vi "OldCombinedPythonIDE.vi"(7 "Python version":string="3.9", 11 "Port":string) -> ()   [LabVIEW 2020]
panel:
  out "Script":string
  in  "Example Codes":u16(ring) items=["backpack.py", "Backpack_Demo.py", "Battery.py", "Buttons.py", "Display.py", "Image.py", "LED.py", "Motion.py", "Motor.py", "Sound.py"]
  out "Library":string="Loading...."
  in  "SPIKE Codes":u16(ring) items=["boot.py", "main.py", "version.py", "rogers.py", "backpack.py"]
  out "S_Library":string="Loading..."
  in  "Name":string="code.py"
  in  "Save SPIKE":bool
  in  "Save PC":bool
  in  "Python Code":string
  out "Console":string
  in  "stop":bool
  in  "Ctrl C":bool
  in  "run":bool
  # "PyVIEW IDE\nversion 0.1b01"
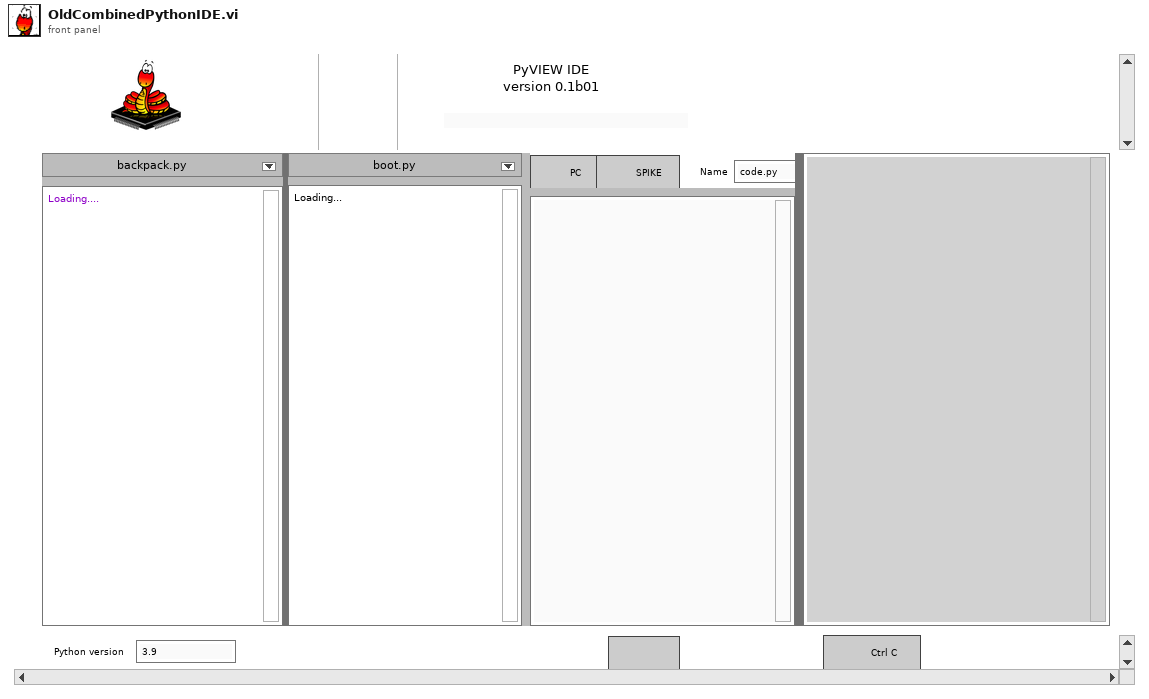
[diagram p1: front panel]
types:
  T1 = typedef "PythonCtrl.ctl" = cluster{"session":refnum<k35>, "PyPath":path, "Processor":enum16{"SPIKE", "Pi", "Pi_ssh"}}
  T2 = typedef "eventvkey.ctl" = enum16{"ASCII", "Enter", "Return", "Shift", "Ctrl", "Alt", "Cmd", "Opt", "Caps", "NumLock", "Clear", "Break", "Up", "Down", "Left", "Right", "Insert", "Delete", "Home", "End", "PageUp", "PageDown", "Escape", "Help", "Pause", "ScrollLock", "F1", "F2", "F3", "F4", "F5", "F6", "F7", "F8", "F9", "F10", "F11", "F12", "F13", "F14", "F15", "F16", "F17", "F18", "F19", "F20", "F21", "F22", "F23", "F24", "Play", "VolumeUp", "VolumeDown", "Mute", "Two Byte Char"}
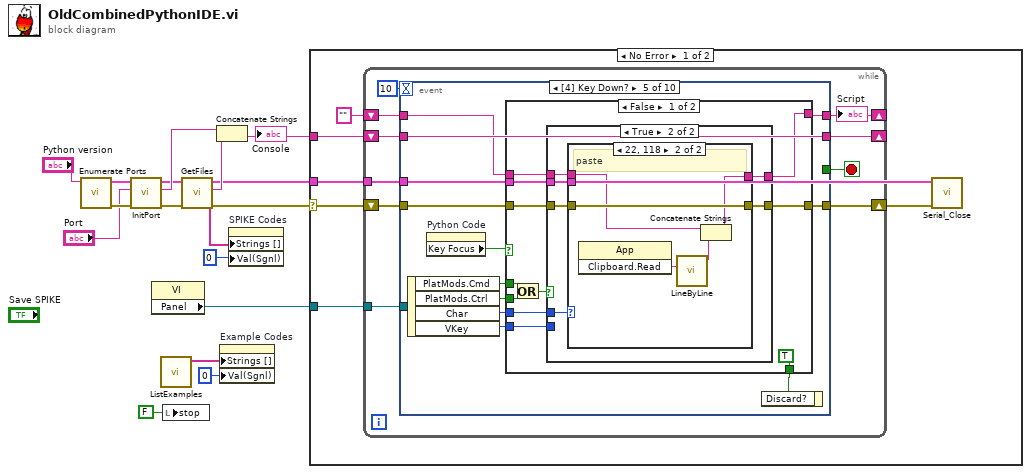
[diagram p0: block diagram]
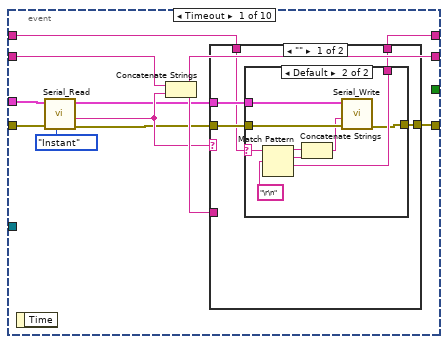
[diagram p2: hidden frame]
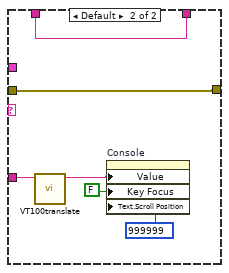
[diagram p4: hidden frame]
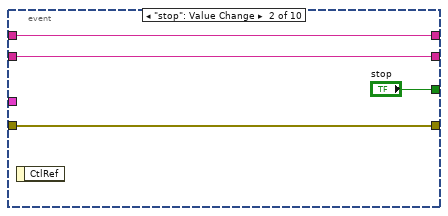
[diagram p5: hidden frame]
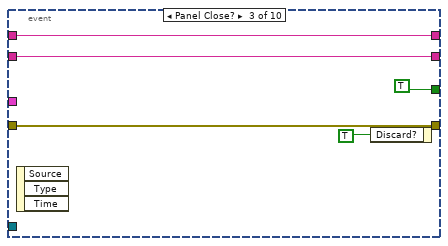
[diagram p6: hidden frame]
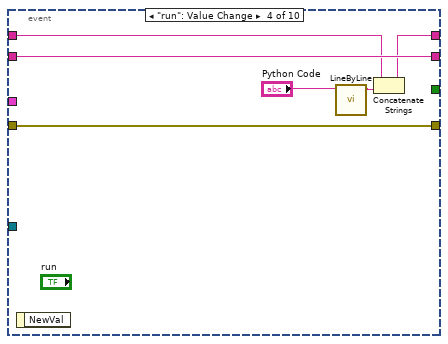
[diagram p7: hidden frame]
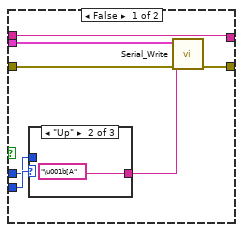
[diagram p8: hidden frame]
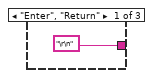
[diagram p9: hidden frame]
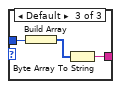
[diagram p10: hidden frame]
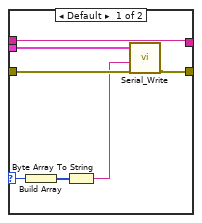
[diagram p11: hidden frame]
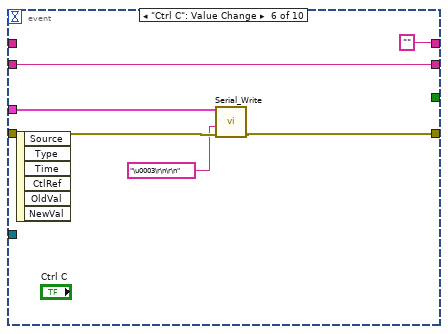
[diagram p14: hidden frame]
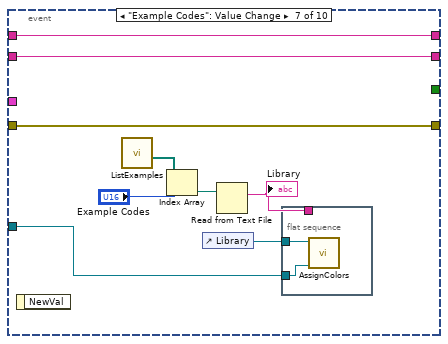
[diagram p15: hidden frame]
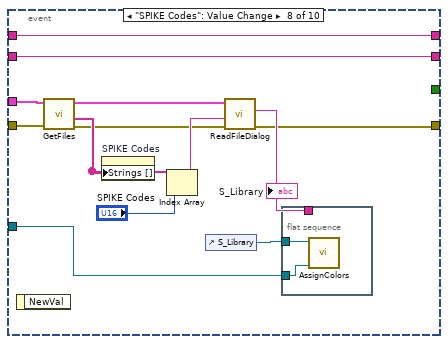
[diagram p16: hidden frame]
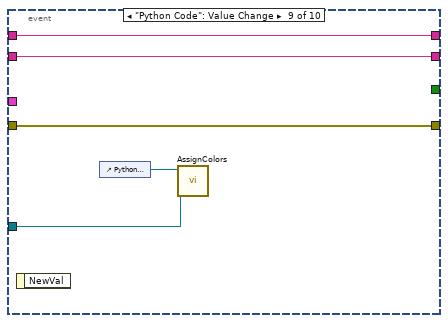
[diagram p17: hidden frame]
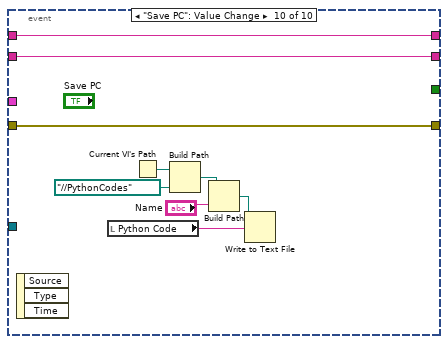
[diagram p18: hidden frame]
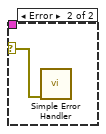
[diagram p19: hidden frame]
diagram:
  n1 = call "Enumerate Ports.vi"("Python version"="Python version") -> ("error out"=w15:errorcluster, "Python"=w9:T1)  [unwired: 6 in, 3 out]
  n2 = call "InitPort.vi"("error in (no error)"=w15, "Port"="Port", "Python"=w9) -> ("error out"=w7:errorcluster, "Console"=w8:string, "Python out"=w4:T1)  [unwired: 6 in]
  n3 = property class="VI"() -> ("Panel"=w10:refnum<vi>)  [unwired: 2 in, 2 out]
  n4 = call "ListExamples.vi"() -> ("filenames"=w11:string[])  [unwired: 7 in, 4 out]
  n5 = local write "stop"(FALSE ("stop")) -> ()
  n6 = call "GetFiles.vi"("error in (no error)"=w7, "Python"=w4) -> ("error out"=w6:errorcluster, "Python files"=w3:string[], "String"=w5:string)  [unwired: 6 in, 1 out]
  n7 = Concatenate Strings(w8, w5) -> (w1:string)
  "Console" <- w1
  n8 = property on="Example Codes" class="Ring (strict)"("Strings []"=w11, "Val(Sgnl)"=u16 0 ("Value (Signaling)")) -> ()  [unwired: 2 in, 2 out]
  n9 = property on="SPIKE Codes" class="Ring (strict)"("Strings []"=w3, "Val(Sgnl)"=u16 0 ("Value (Signaling)")) -> ()  [unwired: 2 in, 2 out]
  n10 = case shown="No Error" w6 {
    selector: w6 -> [w21 w181]
    tunnel: w10 -> [w22 _]
    tunnel: w1 -> [w19 _]
    tunnel: w4 -> [w18 _]
    frame No Error {
      n11 = while {
        shift-right: [w31] -> _
        shift-left: w19 -> [w32]
        shift-right: [w27] -> w17
        shift-left: w21 -> [w28]
        tunnel: w22 -> [w26]
        shift-right: [w24] -> _
        shift-left: "" -> [w25]
        tunnel: w18 -> [w23]
        stop <- w30 stop-if-true
        n12 = event shown="[4] Key Down?" {
          selector: _ -> [_ _ _ _ _ _ _ _ _ _]
          dyn-events: _ -> [_ _ _ _ _ _ _ _ _ _]
          timeout: 10 -> [_ _ _ _ _ _ _ _ _ _]
          tunnel: w23 -> [w34 _ _ _ w91 w140 _ w157 _ _]
          tunnel: w32 -> [w42 w67 w73 w79 w90 w141 w147 w164 w171 w179]
          tunnel: [w41 w67 w73 w79 w90 w141 w147 w164 w171 w179] -> w31
          tunnel: [_ "stop" TRUE ("stop") _ _ _ _ _ _ _] -> w30
          tunnel: w28 -> [w37 w66 w72 w78 w84 w139 w146 w159 w170 w178]
          tunnel: [w40 w66 w72 w78 w85 w137 w146 w153 w170 w178] -> w27
          tunnel: w26 -> [_ _ _ _ _ _ w145 w163 w168 _]
          tunnel: [w39 w65 w69 w76 w80 "" w142 w162 w167 w180] -> w24
          tunnel: w25 -> [w38 w65 w69 w77 w81 _ w142 w162 w167 w180]
          event Timeout {
            n13 = event-data() -> ()  [unwired: 1 in, 1 out]
            n14 = call "Serial_Read.vi"("Task"=enum16{"Instant", "All"}."Instant", "error in (no error)"=w37, "Python"=w34) -> ("error out"=w35:errorcluster, "Text read"=w36:string)  [unwired: 7 in]
            n15 = Concatenate Strings(w42, w36) -> (w41:string)
            n16 = case shown="\"\"" w36 {
              tunnel: w41 -> [_ w64]
              tunnel: w35 -> [w46 w60]
              tunnel: [w45 w60] -> w40
              tunnel: w38 -> [w43 w59]
              tunnel: [w47 w59] -> w39
              tunnel: w34 -> [w44 _]
              frame "" {
                n17 = case shown="Default" w43 {
                  selector: w43 -> [w49 w50]
                  tunnel: [w49 w58] -> w47
                  tunnel: w46 -> [w48 w54]
                  tunnel: [w48 w53] -> w45
                  tunnel: w44 -> [_ w51]
                  frame "" {
                  }
                  frame Default {
                    n18 = Match Pattern(string=w50, regular expression="\r\n") -> (before substring=w56:string, match substring=w55:string, after substring=w58:string)  [unwired: 1 in, 1 out]
                    n19 = Concatenate Strings(w56, w55) -> (w52:string)
                    n20 = call "Serial_Write.vi"("error in (no error)"=w54, "Text to write"=w52, "Python"=w51) -> ("error out"=w53:errorcluster)  [unwired: 8 in]
                  }
                }
              }
              frame Default {
                n21 = call "VT100translate.vi"("Console"=w64) -> ("Console 2"=w62:string)  [unwired: 10 in]
                n22 = property on="Console" class="Str"("Value"=w62, "Key Focus"=FALSE, "Text.Scroll Position"=u32 999999) -> ()  [unwired: 2 in, 2 out]
              }
            }
          }
          event "stop": Value Change {
            n23 = event-data() -> ()  [unwired: 1 in, 1 out]
          }
          event Panel Close? {
            n24 = event-data() -> ()  [unwired: 1 in, 3 out]
            n25 = event-data("Discard?"=TRUE ("stop")) -> ()  [unwired: 1 in, 1 out]
          }
          event "run": Value Change {
            n26 = event-data() -> ()  [unwired: 1 in, 1 out]
            n27 = call "LineByLine.vi"("Python Code"="Python Code") -> ("result string"=w75:string)  [unwired: 10 in]
            n28 = Concatenate Strings(w77, w75) -> (w76:string)
          }
          event Key Down? {
            n29 = event-data() -> ("PlatMods.Cmd"=w86:bool, "PlatMods.Ctrl"=w87:bool, "Char"=w88:i16, "VKey"=w89:T2)  [unwired: 1 in]
            n30 = property on="Python Code" class="Str"() -> ("Key Focus"=w82:bool)  [unwired: 2 in, 2 out]
            n31 = case shown="False" w82 {
              tunnel: w91 -> [w96 _]
              tunnel: w89 -> [w102 _]
              tunnel: w88 -> [w101 w134]
              tunnel: w87 -> [w100 _]
              tunnel: w86 -> [w99 _]
              tunnel: [w94 w135] -> w85
              tunnel: w84 -> [w95 w135]
              tunnel: [TRUE ("Discard?") _] -> w83
              tunnel: w81 -> [w93 w133]
              tunnel: [w92 w133] -> w80
              frame False {
                n32 = Or(x=w99, y=w100) -> (x .or. y?=w98:bool)
                n33 = case shown="True" w98 {
                  tunnel: w102 -> [w109 _]
                  tunnel: w101 -> [w108 w120]
                  tunnel: w96 -> [w107 w119]
                  tunnel: w95 -> [w106 w118]
                  tunnel: [w104 w117] -> w94
                  tunnel: w93 -> [w103 w116]
                  tunnel: [w103 w115] -> w92
                  frame False {
                    n34 = case shown="\"Up\"" w109 {
                      tunnel: w108 -> [_ _ w114]
                      tunnel: ["\r\n" ("replace string (\"\")") "\u001b[A" ("replace string (\"\")") w112] -> w105
                      frame "Enter", "Return" {
                      }
                      frame "Up" {
                      }
                      frame Default {
                        n35 = Build Array(w114) -> (w113:i16[])
                        n36 = Byte Array To String(unsigned byte array=w113) -> (string=w112:string)
                      }
                    }
                    n37 = call "Serial_Write.vi"("error in (no error)"=w106, "Text to write"=w105, "Python"=w107) -> ("error out"=w104:errorcluster)  [unwired: 8 in]
                  }
                  frame True {
                    n38 = case shown="22, 118" w120 {
                      selector: w120 -> [w126 _]
                      tunnel: w119 -> [w125 _]
                      tunnel: w118 -> [w124 w132]
                      tunnel: [w123 w132] -> w117
                      tunnel: w116 -> [w121 w131]
                      tunnel: [w121 w130] -> w115
                      frame Default {
                        n39 = Build Array(w126) -> (w127:i16[])
                        n40 = Byte Array To String(unsigned byte array=w127) -> (string=w122:string)
                        n41 = call "Serial_Write.vi"("error in (no error)"=w124, "Text to write"=w122, "Python"=w125) -> ("error out"=w123:errorcluster)  [unwired: 8 in]
                      }
                      frame 22, 118 {
                        # "paste"
                        n42 = invoke class="App" method="Clipboard.Read"() -> ("Read Clipbrd"=w129:string)  [unwired: 3 in, 2 out]
                        n43 = call "LineByLine.vi"("Python Code"=w129) -> ("result string"=w128:string)  [unwired: 10 in]
                        n44 = Concatenate Strings(w131, w128) -> (w130:string)
                      }
                    }
                  }
                }
              }
              frame True {
                n45 = case shown="1" w134 {
                  frame 0, Default {
                  }
                  frame 1 {
                  }
                }
              }
            }
            n46 = event-data("Discard?"=w83) -> ()  [unwired: 1 in, 1 out]
          }
          event "Ctrl C": Value Change {
            n47 = event-data() -> ()  [unwired: 1 in, 6 out]
            n48 = call "Serial_Write.vi"("error in (no error)"=w139, "Text to write"="\u0003\r\n\r\n" ("function name"), "Python"=w140) -> ("error out"=w137:errorcluster)  [unwired: 8 in]
          }
          event "Example Codes": Value Change {
            n49 = event-data() -> ()  [unwired: 1 in, 1 out]
            n50 = call "ListExamples.vi"() -> ("Paths"=w149:path[])  [unwired: 7 in, 4 out]
            n51 = Index Array(array=w149, index="Example Codes") -> (element=w148:path)
            n52 = control-ref of="Library"() -> (w144:refnum<vi>)
            n53 = Read from Text File(file (use dialog)=w148) -> (text=w143:string)  [unwired: 3 in, 3 out]
            "Library" <- w143
            n54 = flat-sequence {
              tunnel: w145 -> [w152]
              tunnel: w144 -> [w151]
              tunnel: w143 -> [_]
              frame #0 {
                n55 = call "AssignColors.vi"("Front Panel"=w152, "Code"=w151) -> ()  [unwired: 9 in, 1 out]
              }
            }
          }
          event "SPIKE Codes": Value Change {
            n56 = event-data() -> ()  [unwired: 1 in, 1 out]
            n57 = call "GetFiles.vi"("error in (no error)"=w159, "Python"=w157) -> ("error out"=w154:errorcluster, "Python files"=w158:string[])  [unwired: 6 in, 2 out]
            n58 = property on="SPIKE Codes" class="Ring (strict)"("Strings []"=w158) -> ()  [unwired: 2 in, 2 out]
            n59 = Index Array(array=w158, index="SPIKE Codes") -> (element=w156:string)
            n60 = control-ref of="S_Library"() -> (w160:refnum<vi>)
            n61 = call "ReadFileDialog.vi"("error in (no error)"=w154, "File name"=w156, "Python in"=w157) -> ("error out"=w153:errorcluster, "Console"=w155:string)  [unwired: 7 in]
            "S_Library" <- w155
            n62 = flat-sequence {
              tunnel: w163 -> [w166]
              tunnel: w160 -> [w165]
              tunnel: w155 -> [_]
              frame #0 {
                n63 = call "AssignColors.vi"("Front Panel"=w166, "Code"=w165) -> ()  [unwired: 9 in, 1 out]
              }
            }
          }
          event "Python Code": Value Change {
            n64 = event-data() -> ()  [unwired: 1 in, 1 out]
            n65 = control-ref of="Python Code"() -> (w169:refnum<vi>)
            n66 = call "AssignColors.vi"("Front Panel"=w168, "Code"=w169) -> ()  [unwired: 9 in, 1 out]
          }
          event "Save PC": Value Change {
            n67 = event-data() -> ()  [unwired: 1 in, 3 out]
            n68 = local read "Python Code"() -> (w177:string)
            n69 = Current VI's Path() -> (path=w176:path)
            n70 = Build Path(base path=w176, name or relative path=path "../../PythonCodes") -> (appended path=w174:path)
            n71 = Build Path(base path=w174, name or relative path="Name") -> (appended path=w173:path)
            n72 = Write to Text File(file (use dialog)=w173, text=w177) -> ()  [unwired: 2 in, 3 out]
          }
        }
        "Script" <- w24
      }
      n73 = call "Serial_Close.vi"("error in (no error)"=w17, "Python in"=w18) -> ()  [unwired: 10 in]
    }
    frame Error {
      n74 = call <vilib>:"Simple Error Handler.vi"("error in (no error)"=w181) -> ()  [unwired: 4 in, 5 out]
    }
  }
